vi "Set BrowerController Ref.vi"(8 "error in (no error)":errorcluster, 10 "BrowerController Ref":refnum<class "Message Enqueuer.lvclass">, 11 "ProjectController in":refnum<class "ProjectController.lvclass">) -> (0 "error out":errorcluster, 3 "ProjectController out":refnum<class "ProjectController.lvclass">)   [LabVIEW 2015, in "ProjectController.lvclass"]
uses:
  ProjectController.lvclass
  <vilib>/ActorFramework/Message Enqueuer/Message Enqueuer.lvclass
  ProjectController.lvclass/ProjectController.ctl
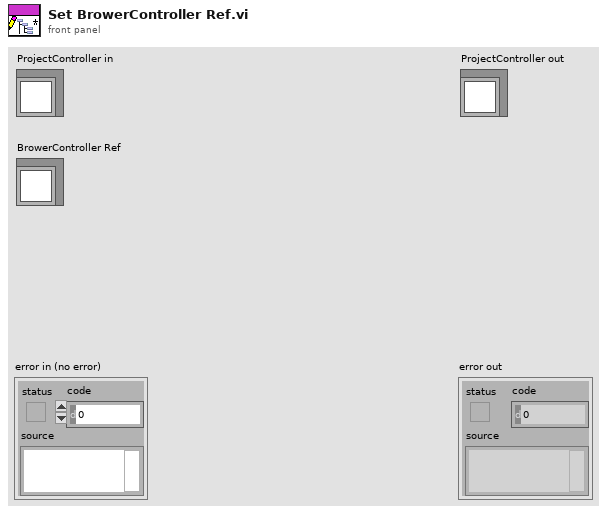
[diagram p1: front panel]
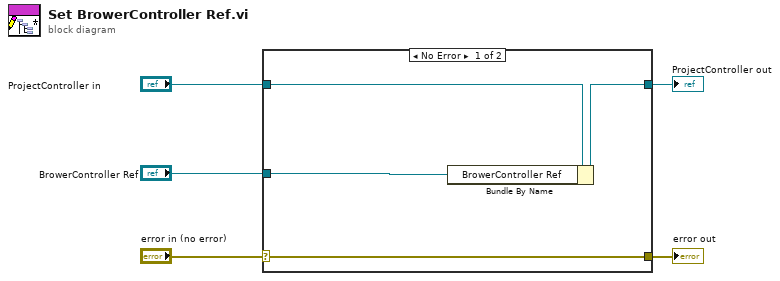
[diagram p0: block diagram]
diagram:
  n1 = case shown="No Error" "error in (no error)" {
    selector: "error in (no error)" -> [w9 w10]
    tunnel: [w9 w10] -> w4
    tunnel: [w7 w11] -> w2
    tunnel: "ProjectController in" -> [w8 w11]
    tunnel: "BrowerController Ref" -> [w6 _]
    frame No Error {
      n2 = Bundle By Name(cluster=w8, "BrowerController Ref"=w6) -> (w7:refnum<class "ProjectController.lvclass">)
    }
    frame Error {
    }
  }
  "error out" <- w4
  "ProjectController out" <- w2
